vi "QueryNetworkSettings.vi"(8 "error in (no error)":errorcluster) -> (0 "error out":errorcluster)   [LabVIEW 2017, in "SystemInfoProcess.lvlib"]
uses:
  <vilib>/addons/SystemInfoProcess/SystemInfoProcess.lvlib
  <vilib>/addons/PointValueMap/PointValueMap.lvlib
  <vilib>/nisyscfg/nisyscfg.lvlib
  <resource>/objmgr/niflexriosae.rc
  <resource>/objmgr/nicriosae.rc
  <vilib>/addons/SystemInfoProcess/controls/NetworkAdapterSettings.ctl
  <vilib>/nisyscfg/Close (Filter).vi
  <vilib>/nisyscfg/Close (Hardware).vi
  <vilib>/nisyscfg/Find Hardware.vi
  <vilib>/addons/PointValueMap/subVIs/Point_Write_variant.vi
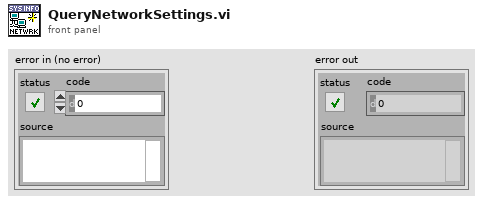
[diagram p1: front panel]
types:
  T1 = typedef "SystemInfoProcess.lvlib/NetworkAdapterSettings.ctl" = cluster{"Adapter Mode":u32, "IsPrimary":bool, "MACAddr":string, "IP Address Request Mode":u32, "IPAddr":string, "SubnetMask":string, "Gateway":string, "DNSServer":string, "Alias":string}
  T2 = typedef "PointValueMap.lvlib/PointMap.ctl" = refnum<data-value>
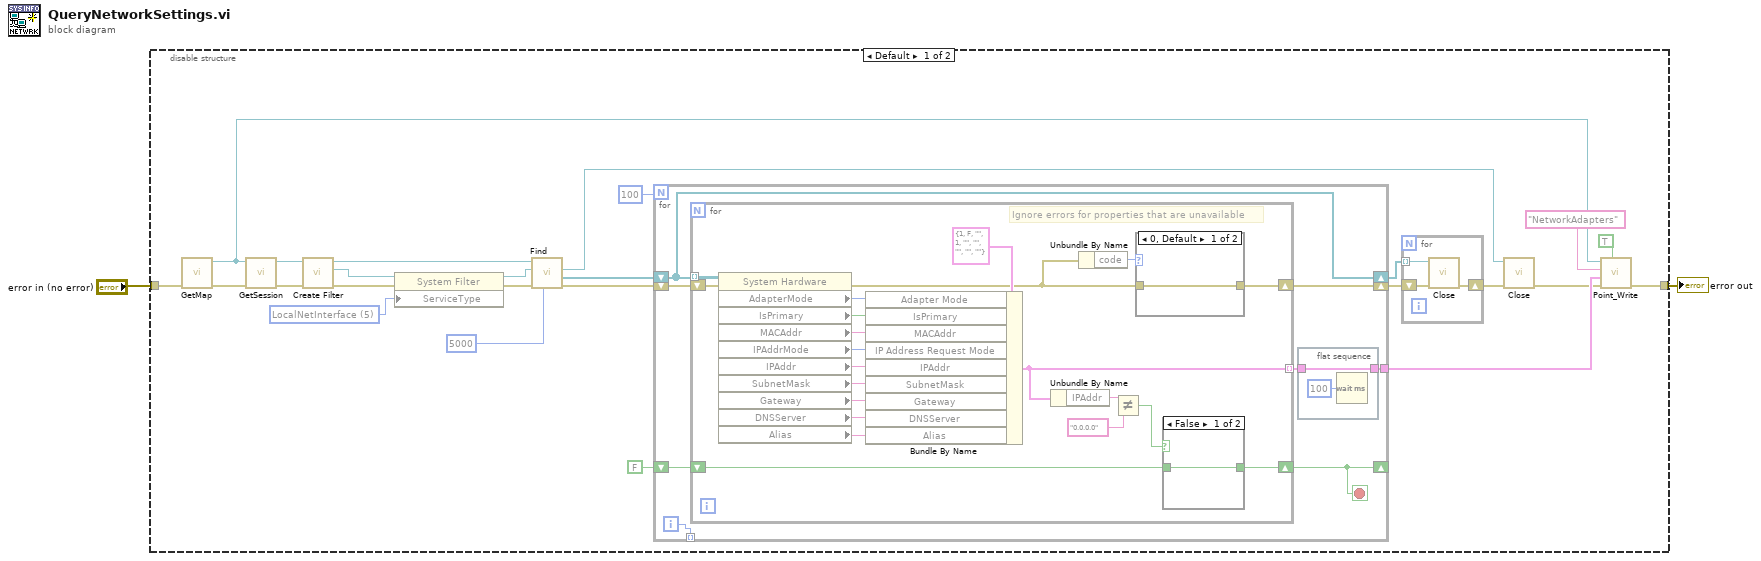
[diagram p0: block diagram]
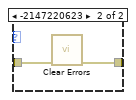
[diagram p3: hidden frame]
diagram:
  n1 = disable-structure shown="Default" {
    disable-tunnel: "error in (no error)" -> [w12 w67]
    disable-tunnel: [w26 w67] -> w1
    frame condition #0 {
      w24 = u32 5 items=["mDnsNiTcp", "mDnsNiRealtime", "mDnsNiSysapi", "mDnsNiHttp", "LocalSystem", "LocalNetInterface", "LocalTimeKeeper", "LocalTimeSource", "mDnsLxi"] ("Service Type")
      n2 = call <vilib>:"GetMap.vi"("error in (no error)"=w12) -> ("error out"=w13:errorcluster, "SystemInfoMap"=w9:T2)  [unwired: 9 in]
      n3 = call <vilib>:"GetSession.vi"("error in (no error)"=w13, "map"=w9) -> ("error out"=w11:errorcluster, "session"=w10:refnum<k21>)  [unwired: 8 in]
      n4 = call <vilib>:"Create Filter.vi"("error in (no error)"=w11, "Session in"=w10) -> ("error out"=w23:errorcluster, "Filter out"=w25:refnum<k20>, "Session out"=w21:refnum<k21>)  [unwired: 7 in]
      n5 = property class="System Filter"(reference=w25, error in=w23, "ServiceType"=w24) -> (reference out=w20:refnum<k20>, error out=w22:errorcluster)
      n6 = call-poly <vilib>:"Find.vi"("Remote Timeout (300,000 ms)"=u32 5000 ("Timeout (milliseconds)"), "error in (no error)"=w22, "Filter in"=w20, "Session in"=w21) -> ("error out"=w18:errorcluster, "Resources out"=w19:refnum<k20>[], "Filter out"=w17:refnum<k20>)  [unwired: 4 in, 1 out]
      n7 = for {
        N: 100 -> [_]
        tunnel: [w34] -> w15
        shift-right: [w37] -> w6
        shift-left: w18 -> [w38]
        shift-right: [w36] -> _
        shift-left: FALSE -> [w33]
        tunnel: [w32] -> _ mode=indexing
        shift-right: [w31] -> w4
        shift-left: w19 -> [w31]
        i -> [w32]
        stop <- w36 stop-if-true
        n8 = for {
          tunnel: w31 -> [w60] mode=indexing
          shift-right: [w50] -> w37
          shift-left: w38 -> [w61]
          tunnel: [w47] -> w35 mode=indexing
          shift-right: [w42] -> w36
          shift-left: w33 -> [w43]
          # "Ignore errors for properties that are unavailable"
          n9 = property class="System Hardware"(reference=w60, error in=w61) -> (error out=w41:errorcluster, "AdapterMode"=w59:u32, "IsPrimary"=w58:bool, "MACAddr"=w57:string, "IPAddrMode"=w56:u32, "IPAddr"=w55:string, "SubnetMask"=w54:string, "Gateway"=w53:string, "DNSServer"=w52:string, "Alias"=w49:string)  [unwired: 1 out]
          n10 = Bundle By Name(cluster=T1 {"Adapter Mode"=1, "IsPrimary"=FALSE, "MACAddr"="", "IP Address Request Mode"=1, "IPAddr"="", "SubnetMask"="", "Gateway"="", "DNSServer"="", "Alias"=""} ("Network Adapter Settings"), "Adapter Mode"=w59, "IsPrimary"=w58, "MACAddr"=w57, "IP Address Request Mode"=w56, "IPAddr"=w55, "SubnetMask"=w54, "Gateway"=w53, "DNSServer"=w52, "Alias"=w49) -> (w47:T1)
          n11 = Unbundle By Name(w47) -> ("IPAddr"=w46:string)
          n12 = Unbundle By Name(w41) -> ("code"=w51:i32)
          n13 = Not Equal?(x=w46, y="0.0.0.0") -> (x != y?=w44:bool)
          n14 = case shown="0, Default" w51 {
            tunnel: [w64 w66] -> w50
            tunnel: w41 -> [w64 w65]
            frame 0, Default {
            }
            frame -2147220623 {
              n15 = call <vilib>:"Clear Errors.vi"("error in (no error)"=w65) -> ("error out"=w66:errorcluster)  [unwired: 5 in, 1 out]
            }
          }
          n16 = case shown="False" w44 {
            selector: w44 -> [_ w63]
            tunnel: w43 -> [w62 _]
            tunnel: [w62 w63] -> w42
            frame False {
            }
            frame True {
            }
          }
        }
        n17 = flat-sequence {
          tunnel: w35 -> [w40]
          tunnel: [w40] -> w34
          frame #0 {
            n18 = Wait (ms)(milliseconds to wait=u32 100) -> ()  [unwired: 1 out]
          }
        }
      }
      n19 = for {
        shift-right: [w29] -> w5
        shift-left: w6 -> [w30]
        tunnel: w4 -> [w28] mode=indexing
        n20 = call-poly <vilib>:"Close.vi"("error in (no error)"=w30, "Resource in"=w28) -> ("error out"=w29:errorcluster)  [unwired: 9 in]
      }
      n21 = call-poly <vilib>:"Close.vi"("error in (no error)"=w5, "Filter in"=w17) -> ("error out"=w3:errorcluster)  [unwired: 9 in]
      n22 = call-poly <vilib>:"Point_Write.vi"("Auto Create?"=TRUE, "Error In"=w3, "Value"=w15, "Tag"="NetworkAdapters", "Map"=w9) -> ("Error Out"=w26:errorcluster)  [unwired: 5 in, 1 out]
    }
    frame condition #1 (active) {
    }
  }
  "error out" <- w1
